vi "Bisect Angle (array).vi"(7 "angle units":T1 items=["radian in, radian out", "radian in, degree out", "degree in, degree out", "degree in, radian out"], 9 "angle bisector range":T2=1 items=["none", "-180 to 180 (-pi to pi)", "0 to 360 (0 to 2pi)"], 10 "End Angle":dbl[](array[numeric]), 11 "Start Angle":dbl[](array[numeric])) -> (0 "error":i32, 3 "Angle Bisector":dbl[](array[numeric]))   [LabVIEW 2017, in "NI_AAL_Angle.lvlib"]
doc: "Calculates the angle that bisects the start angle and the end angle into two equal parts.\n\nWire data to any of the angle inputs to determine the polymorphic instance to use or manually select the instance."
uses:
  <vilib>/Analysis/NI_AAL_Angle.lvlib
  <vilib>/Analysis/coordinate.llb/Angle Range (Degree).ctl
  <vilib>/Analysis/coordinate.llb/Angle Units.ctl
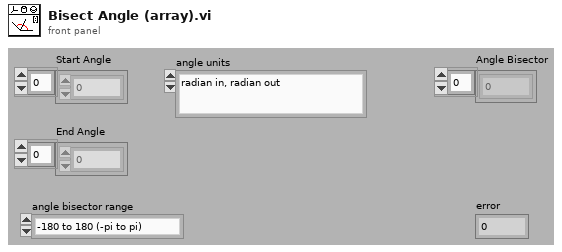
[diagram p1: front panel]
types:
  T1 = typedef "NI_AAL_Angle.lvlib/Angle Units.ctl" = i32
  T2 = typedef "NI_AAL_Angle.lvlib/Angle Range (Degree).ctl" = u16
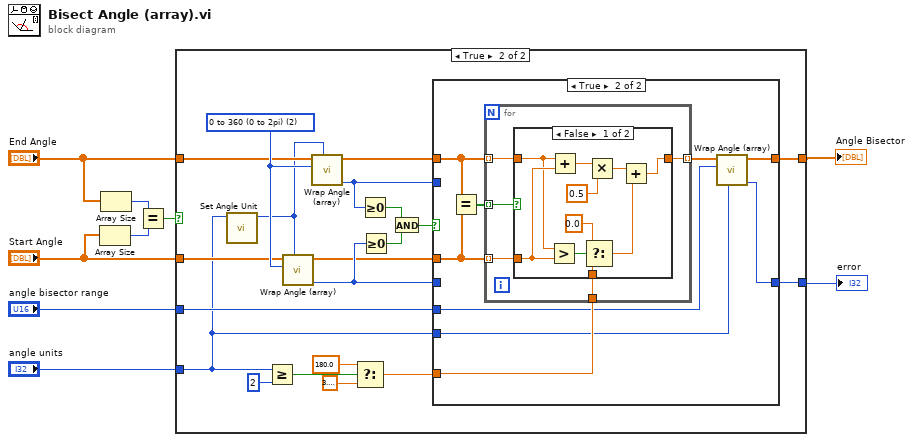
[diagram p0: block diagram]
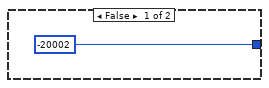
[diagram p2: hidden frame]
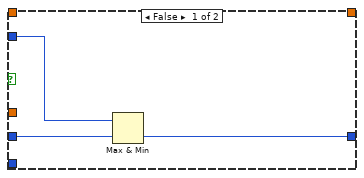
[diagram p3: hidden frame]
diagram:
  n1 = Array Size(array="Start Angle") -> (size(s)=w8:i32)
  n2 = Array Size(array="End Angle") -> (size(s)=w9:i32)
  n3 = Equal?(x=w9, y=w8) -> (x = y?=w3:bool)
  n4 = case shown="True" w3 {
    tunnel: [-20002 ("error") w24] -> w4
    tunnel: "angle bisector range" -> [_ w21]
    tunnel: "angle units" -> [_ w12]
    tunnel: "End Angle" -> [_ w15]
    tunnel: "Start Angle" -> [_ w14]
    tunnel: [_ w13] -> w5
    frame False {
    }
    frame True {
      w30 = T2 2 items=["none", "-180 to 180 (-pi to pi)", "0 to 360 (0 to 2pi)"] ("angle range")
      n5 = call <vilib>:"Set Angle Unit.vi"("angle units in"=w12) -> ("angle units out"=w11:T1)  [unwired: 10 in]
      n6 = Greater Or Equal?(x=w12, y=2) -> (x >= y?=w19:bool)
      n7 = call <vilib>:"Wrap Angle (array).vi"("angle units"=w11, "angle range"=w30, "Angle In"=w14) -> ("error"=w25:i32, "Angle Out"=w22:dbl[])  [unwired: 7 in]
      n8 = call <vilib>:"Wrap Angle (array).vi"("angle units"=w11, "angle range"=w30, "Angle In"=w15) -> ("error"=w26:i32, "Angle Out"=w23:dbl[])  [unwired: 7 in]
      n9 = Select(t=180.0, s=w19, f=3.141592653589793) -> (s? t:f=w16:dbl)
      n10 = Greater Or Equal To 0?(x=w26) -> (x >= 0?=w29:bool)
      n11 = Greater Or Equal To 0?(x=w25) -> (x >= 0?=w28:bool)
      n12 = And(x=w29, y=w28) -> (x .and. y?=w27:bool)
      n13 = case shown="True" w27 {
        tunnel: w26 -> [w33 _]
        tunnel: w25 -> [w32 _]
        tunnel: [w31 w35] -> w24
        tunnel: [_ w37] -> w13
        tunnel: w23 -> [_ w41]
        tunnel: w22 -> [_ w40]
        tunnel: w21 -> [_ w36]
        tunnel: w12 -> [_ w34]
        tunnel: w16 -> [_ w39]
        frame False {
          n14 = Max & Min(x=w33, y=w32) -> (min(x,y)=w31:i32)  [unwired: 1 out]
        }
        frame True {
          n15 = Equal?(x=w41, y=w40) -> (x = y?=w42:bool[])
          n16 = for {
            tunnel: w42 -> [w47] mode=indexing
            tunnel: w41 -> [w46] mode=indexing
            tunnel: [w45] -> w38 mode=indexing
            tunnel: w40 -> [w44] mode=indexing
            tunnel: w39 -> [w43]
            n17 = case shown="False" w47 {
              tunnel: w46 -> [w54 w58]
              tunnel: [w48 w58] -> w45
              tunnel: w44 -> [w55 _]
              tunnel: w43 -> [w51 _]
              frame False {
                n18 = Greater?(x=w54, y=w55) -> (0:w53:bool)
                n19 = Add(x=w54, y=w55) -> (x+y=w57:dbl)
                n20 = Select(t=0.0, s=w53, f=w51) -> (s? t:f=w49:dbl)
                n21 = Multiply(x=w57, y=0.5) -> (x*y=w50:dbl)
                n22 = Add(x=w50, y=w49) -> (x+y=w48:dbl)
              }
              frame True {
              }
            }
          }
          n23 = call <vilib>:"Wrap Angle (array).vi"("angle units"=w34, "angle range"=w36, "Angle In"=w38) -> ("error"=w35:i32, "Angle Out"=w37:dbl[])  [unwired: 7 in]
        }
      }
    }
  }
  "Angle Bisector" <- w5
  "error" <- w4
